vi "configuration_file.vi"() -> ()   [LabVIEW 2017]
uses:
  <vilib>/Utility/config.llb/Read Key (String).vi
  <vilib>/Utility/config.llb/NI_LVConfig.lvlib
panel:
  out "value":string
  out "key names":string[](array[string])
  out "section names":string[](array[string])
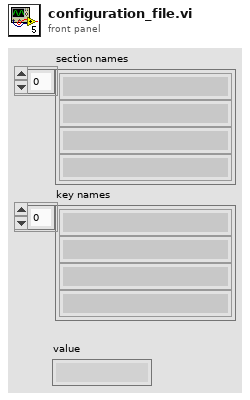
[diagram p1: front panel]
types:
  T1 = typedef "NI_LVConfig.lvlib/Config Data RefNum.ctl" = refnum<k1>
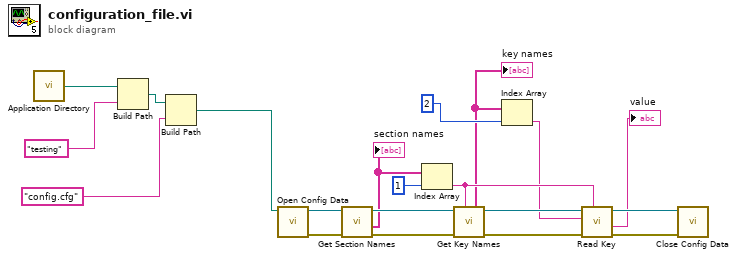
[diagram p0: block diagram]
diagram:
  n1 = call <vilib>:"Application Directory.vi"() -> ("Application Directory"=w20:path)
  n2 = Build Path(base path=w20, name or relative path="testing") -> (appended path=w16:path)
  n3 = Build Path(base path=w16, name or relative path="config.cfg") -> (appended path=w14:path)
  n4 = call <vilib>:"Open Config Data.vi"("configuration file path"=w14) -> ("error out"=w18:errorcluster, "refnum"=w17:T1)  [unwired: 8 in, 1 out]
  n5 = call <vilib>:"Get Section Names.vi"("error in (no error)"=w18, "refnum"=w17) -> ("error out"=w13:errorcluster, "section names"=w11:string[], "refnum out"=w12:T1)  [unwired: 7 in]
  "section names" <- w11
  n6 = Index Array(array=w11, index=1) -> (element=w5:string)
  n7 = call <vilib>:"Get Key Names.vi"("section"=w5, "error in (no error)"=w13, "refnum"=w12) -> ("error out"=w9:errorcluster, "key names"=w3:string[], "refnum out"=w8:T1)  [unwired: 5 in, 1 out]
  "key names" <- w3
  n8 = Index Array(array=w3, index=2) -> (element=w2:string)
  n9 = call-poly <vilib>:"Read Key.vi"("section"=w5, "error in (no error)"=w9, "key"=w2, "refnum"=w8) -> ("error out"=w6:errorcluster, "value"=→"value":string, "refnum out"=w7:T1)  [unwired: 4 in, 1 out]
  n10 = call <vilib>:"Close Config Data.vi"("error in (no error)"=w6, "refnum"=w7) -> ()  [unwired: 8 in, 2 out]
